vi "Simple Add.vi"() -> ()   [LabVIEW 2018]
panel:
  in  "C":dbl
  out "A+B+C":dbl
  in  "B":dbl
  in  "A":dbl
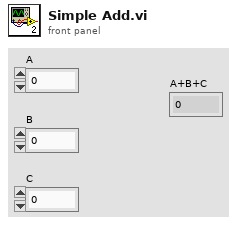
[diagram p1: front panel]
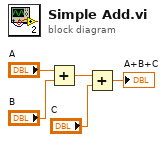
[diagram p0: block diagram]
diagram:
  n1 = Add(x="A", y="B") -> (x+y=w3:dbl)
  n2 = Add(x=w3, y="C") -> (x+y=→"A+B+C":dbl)
